vi "rszvl Configure Source Power.vi"(8 "error in (no error)":errorcluster, 9 "Source Power (-10.0)":dbl=-10.0 format="%^.3e", 10 "Channel (1)":i32=1, 11 "VISA resource name":refnum<visa-resource-name>) -> (0 "error out":errorcluster, 3 "VISA resource name out":refnum<visa-resource-name>)   [LabVIEW 2014]
doc: "This VI defines the power of the internal signal source (channel power). The setting is valid for all sweep types.\n\nAttribute(s):\nRSZVL_ATTR_NWA_SOURCE_POWER\n\nRemote-control command(s):\nSOURce<Ch>:POWer<Pt>[:LEVel][:IMMediate][:AMPlitude]"
uses:
  Instance           2 36Saved   rszvl Configure Source Power .vi
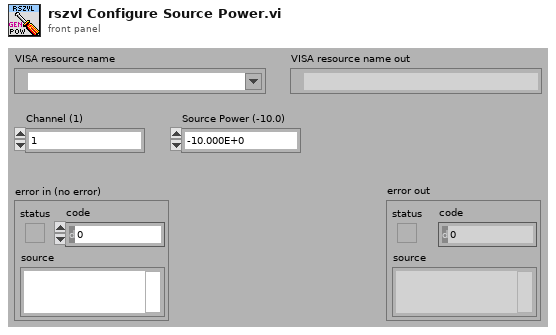
[diagram p1: front panel]
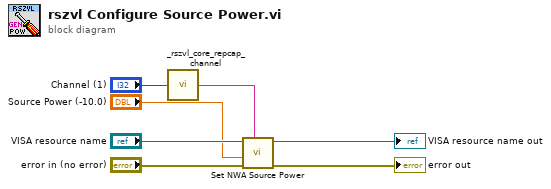
[diagram p0: block diagram]
diagram:
  n1 = call "_rszvl_core_repcap_channel.vi"("Channel"="Channel (1)") -> ("Rep cap"=w7:string)
  n2 = call "Set NWA Source Power"("Repeated Capabilities"=w7, "error in (no error)"="error in (no error)", "NWA Source Power (-10.0)"="Source Power (-10.0)", "instrument handle"="VISA resource name") -> ("error out"=→"error out":errorcluster, "instrument handle out"=→"VISA resource name out":refnum<visa-resource-name>)  [unwired: 6 in]
